vi "st_Percentiles (scalar).vi"(10 "p":dbl, 11 "x array":dbl[](array[numeric])) -> (0 "error":i32, 3 "percentile":dbl)   [LabVIEW 2010, in "NI_Gmath.lvlib"]
doc: "Computes a value that is greater than <B>p</B> percent of the data values in <B>x array</B>. Wire data to the <B>p</B> input to determine the polymorphic instance to use or manually select the instance."
uses:
  NI_Gmath.lvlib
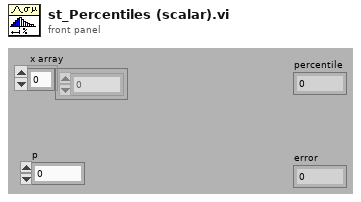
[diagram p1: front panel]
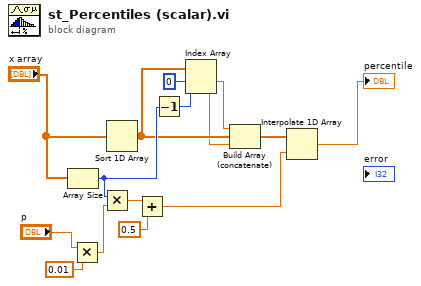
[diagram p0: block diagram]
diagram:
  n1 = Array Size(array="x array") -> (size(s)=w7:i32)
  n2 = Multiply(x="p", y=0.01) -> (x*y=w12:dbl)
  n3 = Multiply(x=w7, y=w12) -> (x*y=w11:dbl)
  n4 = Sort 1D Array(array="x array") -> (sorted array=w5:dbl[])
  n5 = Add(x=w11, y=0.5) -> (x+y=w2:dbl)
  n6 = Decrement(x=w7) -> (x-1=w8:i32)
  n7 = Index Array(array=w5, index #1=0 ("index"), index #2=w8) -> (element #1=w6:dbl, element #2=w4:dbl)
  n8 = Build Array (concatenate)(w6, w5, w4) -> (w3:dbl[])
  n9 = Interpolate 1D Array(1:w2, 2:w3) -> (0:→"percentile":dbl)
